vi "KH_EthernetIP_ReinitConnection.vi"(8 "error in":errorcluster, 11 "address":string) -> (0 "error out":errorcluster, 3 "connection ID":refnum<k5>)   [LabVIEW 2021]
uses:
  KH_EthernetIP_Globals.vi
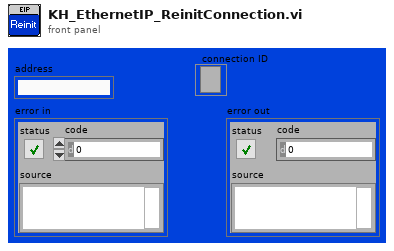
[diagram p1: front panel]
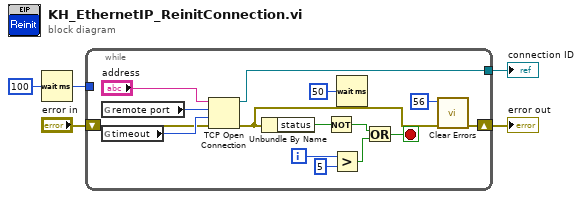
[diagram p0: block diagram]
diagram:
  n1 = Wait (ms)(milliseconds to wait=u32 100) -> (millisecond timer value=w1:u32)
  n2 = while {
    shift-right: [w7] -> w4
    shift-left: "error in" -> [w12]
    tunnel: [w9] -> w3
    tunnel: w1 -> [_]
    i -> [w15]
    stop <- w13 stop-if-true
    n3 = global read "KH_EthernetIP_Globals.vi" "remote port"() -> (w17:u16)
    n4 = global read "KH_EthernetIP_Globals.vi" "timeout"() -> (w18:i32)
    n5 = TCP Open Connection(address="address", remote port or service name=w17, timeout ms (60000)=w18, error in (no error)=w12) -> (connection ID=w9:refnum<k5>, error out=w8:errorcluster)  [unwired: 1 in]
    n6 = Unbundle By Name(w8) -> ("status"=w11:bool)
    n7 = Not(x=w11) -> (.not. x?=w10:bool)
    n8 = Greater?(x=w15, y=5) -> (0:w16:bool)
    n9 = Wait (ms)(milliseconds to wait=u32 50) -> ()  [unwired: 1 out]
    n10 = Or(x=w10, y=w16) -> (x .or. y?=w13:bool)
    n11 = call <vilib>:"Clear Errors.vi"("error in (no error)"=w8, "specific error code to clear (0: all)"=56) -> ("error out"=w7:errorcluster)  [unwired: 4 in, 1 out]
  }
  "error out" <- w4
  "connection ID" <- w3
